vi "I2C Grove 8x8 Matrix LED Custom.vi"() -> ()   [LabVIEW 2020, in "CTI-Scratchpad.lvlib"]
uses:
  CTI-Scratchpad.lvlib
  CTI/Identity.ctl
  CTI-Peripheral/RGB LED Matrix/Grove 2 RGB LED Matrix/Data Types/Colors.ctl
  CTI/Error Reporting.ctl
  CTI/GPIO Number.ctl
  CTI/I2C Number.ctl
  CTI/Session/Session.lvclass
  CTI-Peripheral/RGB LED Matrix/Grove 2 RGB LED Matrix/Grove 2 RGB LED Matrix.lvclass
  CTI/VisaComms/VisaComms.lvclass
  CTI/CTI.lvlib
panel:
  out "Version":string
  in  "Matrix":T1[][](array[typedef])=[[255, 255, 24, 255, 255, 255, 255, 255], [255, 255, 24, 24, 24, 255, 255, 255], [255, 255, 24, 24, 255, 24, 255, 255], [255, 255, 24, 255, 255, 255, 24, 255], [255, 255, 24, 24, 255, 24, 255, 255], [255, 255, 24, 24, 24, 255, 255, 255], [255, 255, 24, 255, 255, 255, 255, 255], [255, 255, 255, 255, 255, 255, 255, 255]] items=["red"=0, "orange"=18, "yellow"=24, "green"=82, "cyan"=127, "blue"=170, "purple"=195, "pink"=220, "white"=254, "black"=255]
  in  "Set Display":bool
  out "LED Colours":u8[][](array[ramp])
  out "Identity":T2
  in  "stop":bool
  in  "Grove Connector":enum16{"I2C0", "I2C1"}(ring)
  out "error out":errorcluster
  in  "Port":refnum<visa-resource-name>="COM4"
  # "https://wiki.seeedstudio.com/Grove-RGB_LED_Matrix_w-Driver/"
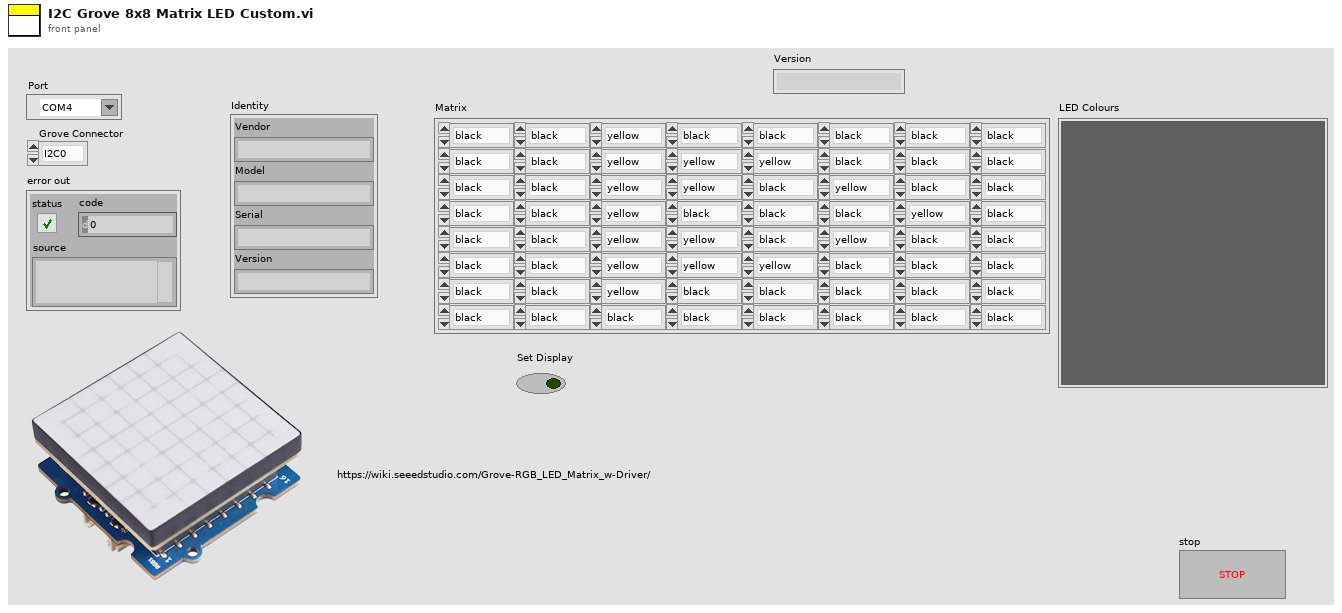
[diagram p1: front panel]
types:
  T1 = typedef "CTI-Peripheral.lvlib/Grove 2 RGB LED Matrix.lvclass/Colors.ctl" = u8
  T2 = typedef "CTI.lvlib/Identity.ctl" = cluster{"Vendor":string, "Model":string, "Serial":string, "Version":string}
  T3 = typedef "CTI.lvlib/Error Reporting.ctl" = enum16{"Minimal", "Moderate", "Full"}
  T4 = typedef "CTI.lvlib/I2C Number.ctl" = i8
  T5 = typedef "CTI.lvlib/GPIO Number.ctl" = i8
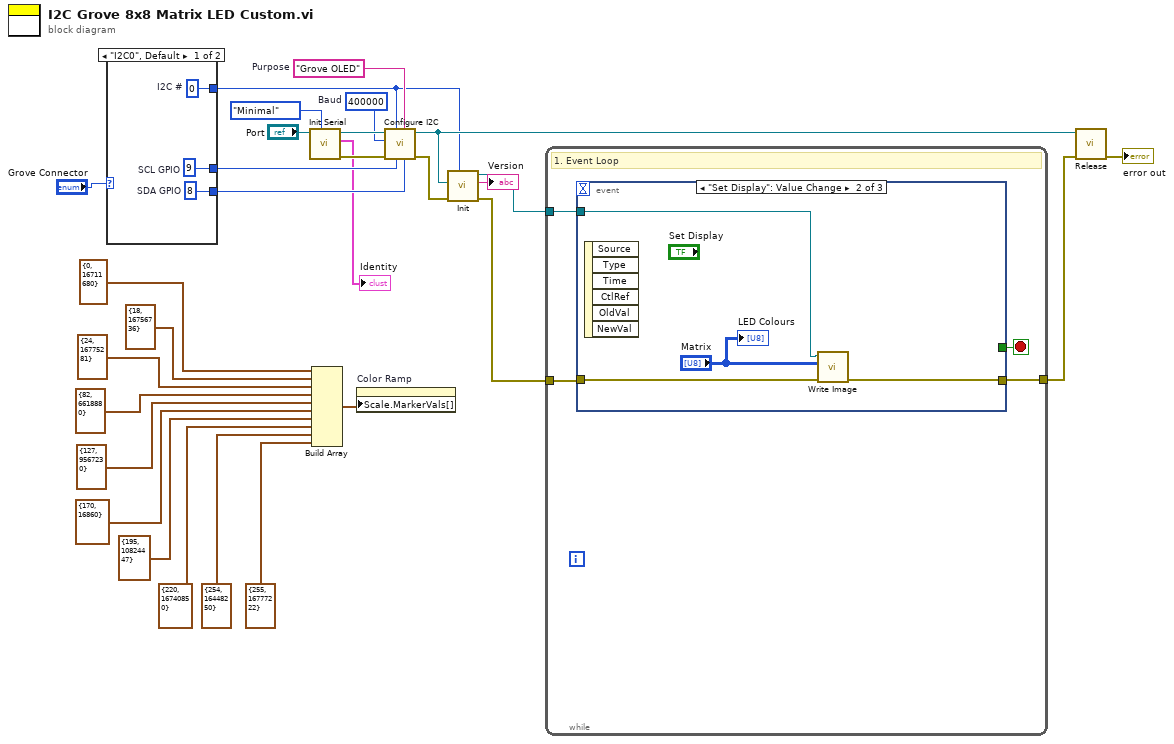
[diagram p0: block diagram]
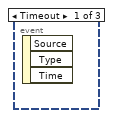
[diagram p2: hidden frame]
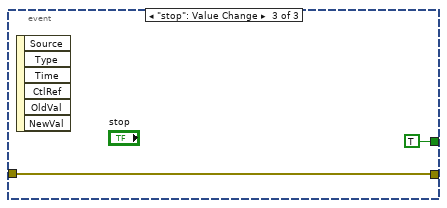
[diagram p3: hidden frame]
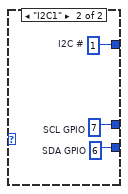
[diagram p4: hidden frame]
diagram:
  w24 = "Grove OLED"  # Purpose
  w25 = u32 400000  # Baud
  n1 = case shown="\"I2C0\", Default" "Grove Connector" {
    tunnel: [w32 w35] -> w20
    tunnel: [w31 w34] -> w19
    tunnel: [w30 w33] -> w18
    frame "I2C0", Default {
      w30 = T4 0  # I2C #
      w31 = T5 8  # SDA GPIO
      w32 = T5 9  # SCL GPIO
    }
    frame "I2C1" {
      w33 = T4 1  # I2C #
      w34 = T5 6  # SDA GPIO
      w35 = T5 7  # SCL GPIO
    }
  }
  n2 = call "Init Serial.vi"("Error Checking (Full)"=Error_Reporting."Minimal", "VISA resource name in"="Port") -> ("error out"=w26:errorcluster, "Identity"=→"Identity":T2, "Session"=w27:refnum<class "Session.lvclass">)  [unwired: 7 in]
  n3 = Build Array(cluster{i32, u32} {0, 16711680}, cluster{i32, u32} {18, 16756736}, cluster{i32, u32} {24, 16775281}, cluster{i32, u32} {82, 6618880}, cluster{i32, u32} {127, 9567230}, cluster{i32, u32} {170, 16860}, cluster{i32, u32} {195, 10824447}, cluster{i32, u32} {220, 16740850}, cluster{i32, u32} {254, 16448250}, cluster{i32, u32} {255, 16777222}) -> (w11:cluster{i32, u32}[])
  n4 = property on="Color Ramp" class="ColRmp (strict)"("Scale.MarkerVals[]"=w11) -> ()  [unwired: 2 in, 2 out]
  n5 = call "Configure I2C.vi"("SDA GPIO"=w19, "Purpose (\"I2C\")"=w24, "SCL GPIO"=w20, "I2C #"=w18, "error in (no error)"=w26, "Baud"=w25, "Session in"=w27) -> ("error out"=w23:errorcluster, "Session out"=w22:refnum<class "Session.lvclass">)  [unwired: 3 in]
  n6 = call "Init.vi"("I2C #"=w18, "error in (no error)"=w23, "Session In"=w22) -> ("error out"=w16:errorcluster, "Version"=→"Version":string, "Grove 2 RGB LED Matrix Out"=w13:refnum<class "Grove 2 RGB LED Matrix.lvclass">)  [unwired: 6 in]
  n7 = while {
    tunnel: w16 -> [w38]
    tunnel: [w37] -> w15
    tunnel: w13 -> [w39]
    stop <- w36 stop-if-true
    # "1. Event Loop"
    n8 = event shown="[1] \"Set Display\": Value Change" {
      selector: _ -> [_ _ _]
      dyn-events: _ -> [_ _ _]
      timeout: _ -> [_ _ _]
      tunnel: w39 -> [_ w41 _]
      tunnel: w38 -> [_ w43 w45]
      tunnel: [_ w42 w45] -> w37
      tunnel: [_ _ TRUE] -> w36
      event Timeout {
        n9 = event-data() -> ()  [unwired: 1 in, 3 out]
      }
      event "Set Display": Value Change {
        n10 = event-data() -> ()  [unwired: 1 in, 6 out]
        n11 = call-dynamic "Write Image.vi"("error in (no error)"=w43, "Matrix"="Matrix", "Grove 2 RGB LED Matrix In"=w41) -> ("error out"=w42:errorcluster)  [unwired: 7 in, 1 out]
        "LED Colours" <- "Matrix"
      }
      event "stop": Value Change {
        n12 = event-data() -> ()  [unwired: 1 in, 6 out]
      }
    }
  }
  n13 = call-dynamic "Release.vi"("error in (no error)"=w15, "Session in"=w22) -> ("error out"=→"error out":errorcluster)  [unwired: 9 in]
